vi "Destroy.vi"(11 "Circular Buffer in":refnum<class "Circular Buffer.lvclass">) -> ()   [LabVIEW 2023, in "d20.lvlib" / "Circular Buffer.lvclass"]
uses:
  Circular Buffer.lvclass
  Node/Node.lvclass
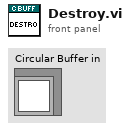
[diagram p1: front panel]
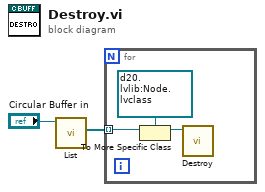
[diagram p0: block diagram]
diagram:
  n1 = call "List.vi"("Circular Buffer in"="Circular Buffer in") -> ("Node List"=w1:refnum<data-value>[])  [unwired: 7 in, 3 out]
  n2 = for {
    tunnel: w1 -> [w5] mode=indexing
    n3 = To More Specific Class(target class=refnum<data-value> refnum ("Data Value Reference in"), reference=w5) -> (specific class reference=w4:refnum<data-value>)  [unwired: 1 in, 1 out]
    n4 = call "Destroy.vi"("Data Value Reference in"=w4) -> ()  [unwired: 11 in]
  }
